vi "LINAKCheckBounds.vi"(0 "MaxExtend":dbl, 1 "AbsRequest":dbl, 2 "MinContract":dbl, 3 "error in (no error)":errorcluster) -> (6 "Request Out":dbl, 8 "error out":errorcluster)   [LabVIEW 2021]
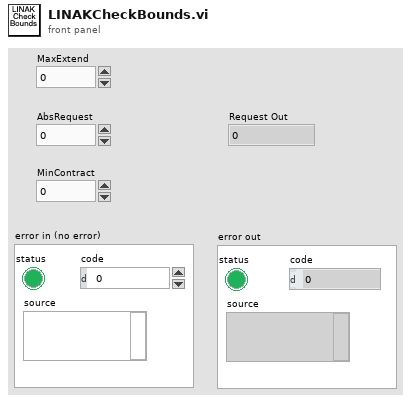
[diagram p1: front panel]
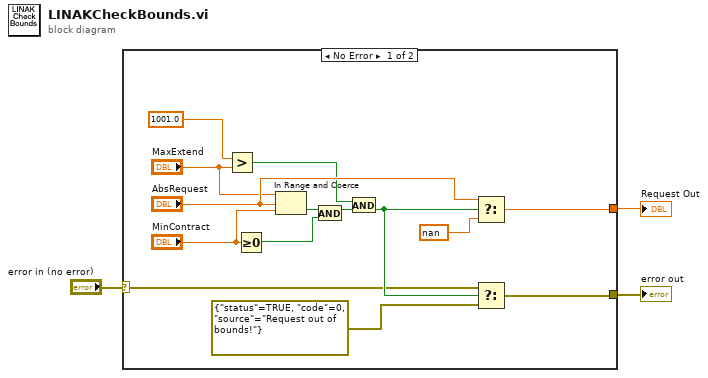
[diagram p0: block diagram]
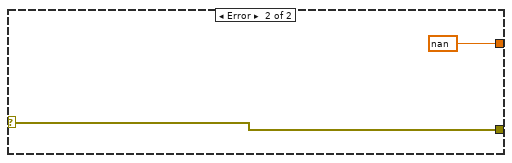
[diagram p2: hidden frame]
diagram:
  n1 = case shown="No Error" "error in (no error)" {
    selector: "error in (no error)" -> [w4 w18]
    tunnel: [w14 w18] -> w2
    tunnel: [w12 nan] -> w1
    frame No Error {
      n2 = Greater?(x=1001.0, y="MaxExtend") -> (0:w8:bool)
      n3 = Greater Or Equal To 0?(x="MinContract") -> (x >= 0?=w6:bool)
      n4 = In Range and Coerce(upper limit="MaxExtend", x="AbsRequest", lower limit="MinContract") -> (In Range?=w15:bool)  [unwired: 1 out]
      n5 = And(x=w15, y=w6) -> (x .and. y?=w7:bool)
      n6 = And(x=w8, y=w7) -> (x .and. y?=w10:bool)
      n7 = Select(t="AbsRequest", s=w10, f=nan) -> (s? t:f=w12:dbl)
      n8 = Select(t=w4, s=w10, f=errorcluster {"status"=TRUE, "code"=0, "source"="Request out of bounds!"}) -> (s? t:f=w14:errorcluster)
    }
    frame Error {
    }
  }
  "error out" <- w2
  "Request Out" <- w1
